vi "read builder target file.vi"(11 "Builder in":refnum<class "Builder.lvclass">) -> (2 "builder target type":refnum<class "NI_AB_API_Build.lvclass">)   [LabVIEW 2024, in "Builder.lvclass"]
uses:
  Builder.lvclass
  Builder.lvclass/Builder.ctl
  <vilib>/AppBuilder/AB_API/Build/NI_AB_API_Build.lvclass
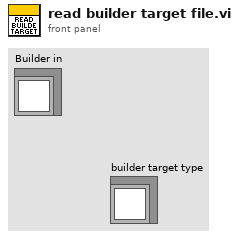
[diagram p1: front panel]
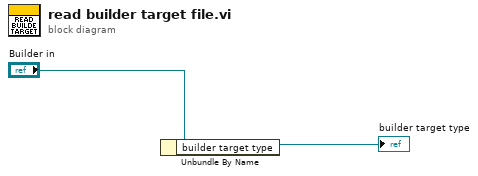
[diagram p0: block diagram]
diagram:
  n1 = Unbundle By Name("Builder in") -> ("builder target type"=→"builder target type":refnum<class "NI_AB_API_Build.lvclass">)
